vi "LockSemaphore.vi"(0 "reference in":refnum<class "VdTcpIP.lvclass">, 2 "LockTimeout(-1)":i32=-1, 5 "error in (no error)":errorcluster) -> (14 "reference out":refnum<class "VdTcpIP.lvclass">, 16 "Locked":bool, 19 "error out":errorcluster)   [LabVIEW 2020, in "VdTcpIP.lvclass"]
uses:
  VdTcpIP.lvclass
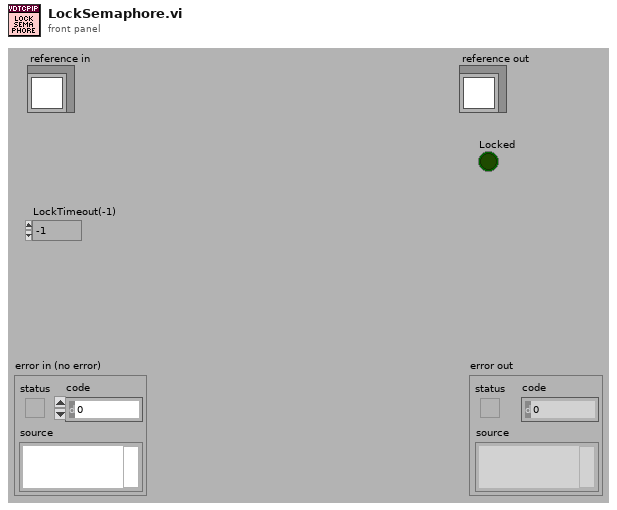
[diagram p1: front panel]
types:
  T1 = typedef "VdTcpIP.lvclass/ObjectAttributes.ctl" = cluster{"IP-Address":string, "Port":u16, "Connection":refnum<k5>, "Listener":refnum<k5>, "ListenerConnection":refnum<k5>, "Listner":bool, "ListnerProcessRunning":bool, "InConnections":refnum<k5>[], "InConnectionsIP":string[], "InConnectionAdded":refnum<notifier>, "RunVIOnNewConnection":variant, "DataToNewConnectionVI":cluster{"ControlName":string, "ControlValue":variant}[], "WebServicesURL_Location(http://...)":string, "WebServicesPostWebPage(*.asmx)":string, "Semaphore":T2, "AutoReConnectTimes":i32, "AutoReConnectInterval(ms)":i32, "ConnectionTimeout":i32}
  T2 = typedef "Semaphore RefNum" = refnum<k1>
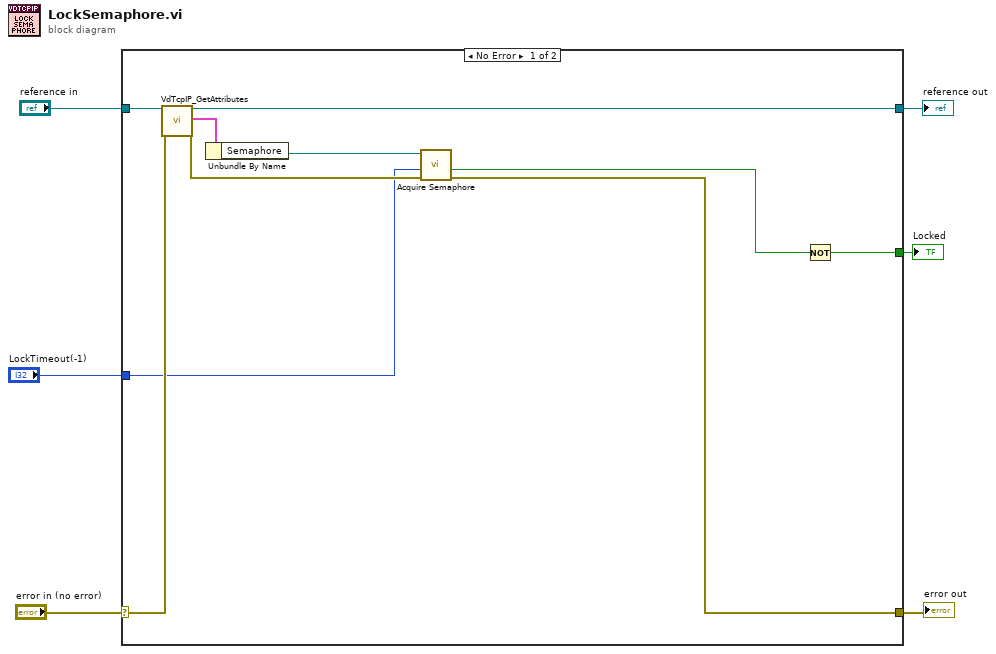
[diagram p0: block diagram]
diagram:
  n1 = case shown="No Error" "error in (no error)" {
    selector: "error in (no error)" -> [w16 w18]
    tunnel: [w11 w18] -> w5
    tunnel: [w14 w17] -> w3
    tunnel: "reference in" -> [w15 w17]
    tunnel: [w9 _] -> w2
    tunnel: "LockTimeout(-1)" -> [w8 _]
    frame No Error {
      n2 = call "VdTcpIP_GetAttributes.vi"("reference in"=w15, "error in (no error)"=w16) -> ("reference out"=w14:refnum<class "VdTcpIP.lvclass">, "Data"=w7:T1, "error out"=w12:errorcluster)  [unwired: 14 in, 1 out]
      n3 = Unbundle By Name(w7) -> ("Semaphore"=w13:T2)
      n4 = call <vilib>:"Acquire Semaphore.vi"("error in (no error)"=w12, "ms timeout (-1)"=w8, "semaphore"=w13) -> ("error out"=w11:errorcluster, "timed out"=w10:bool)  [unwired: 2 in, 1 out]
      n5 = Not(x=w10) -> (.not. x?=w9:bool)
    }
    frame Error {
    }
  }
  "error out" <- w5
  "reference out" <- w3
  "Locked" <- w2
